vi "Ej_2_Verificador_Info.vi"() -> ()   [LabVIEW 2020]
panel:
  out "Nombre confirmado":string
  out "Boolean":bool
  in  "Table Control":string[][](table)
  in  "Contraseña":string
  in  "Nombre":string
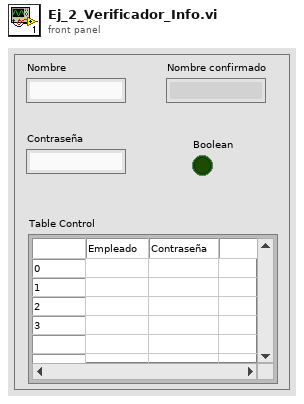
[diagram p1: front panel]
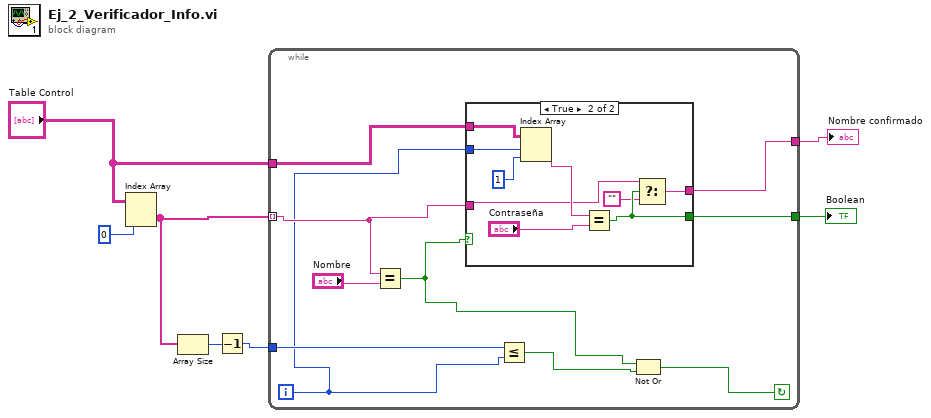
[diagram p0: block diagram]
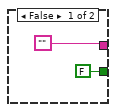
[diagram p2: hidden frame]
diagram:
  n1 = Index Array(array="Table Control", index (col)=0 ("disabled index (col)")) -> (element=w5:string[])  [unwired: 1 in]
  n2 = Array Size(array=w5) -> (size(s)=w7:i32)
  n3 = Decrement(x=w7) -> (x-1=w6:i32)
  n4 = while {
    tunnel: w6 -> [w15]
    tunnel: w5 -> [w13] mode=indexing
    tunnel: [w12] -> w4
    tunnel: [w11] -> w3
    tunnel: "Table Control" -> [w10]
    i -> [w9]
    stop <- w17 continue-if-true
    n5 = Equal?(x=w13, y="Nombre") -> (x = y?=w8:bool)
    n6 = case shown="True" w8 {
      tunnel: w10 -> [_ w22]
      tunnel: w13 -> [_ w25]
      tunnel: [FALSE w24] -> w12
      tunnel: ["" w23] -> w11
      tunnel: w9 -> [_ w21]
      frame False {
      }
      frame True {
        n7 = Index Array(array=w22, index (row)=w21, index (col)=1) -> (element=w26:string)
        n8 = Equal?(x=w26, y="Contraseña") -> (x = y?=w24:bool)
        n9 = Select(t=w25, s=w24, f="") -> (s? t:f=w23:string)
      }
    }
    n10 = Less Or Equal?(x=w15, y=w9) -> (x <= y?=w16:bool)
    n11 = Not Or(1:w16, 2:w8) -> (0:w17:bool)
  }
  "Boolean" <- w4
  "Nombre confirmado" <- w3
